vi "Configure RBW List.vi"(8 "error in (no error)":errorcluster, 9 "Resolution Bandwidth Type List":i32[](array[ring])=[0, 0, 0] items=["Gaussian", "Flattop"], 10 "Resolution Bandwidth List":dbl[](array[numeric])=[1000.0, 1000.0, 1000.0], 11 "VISA resource name":refnum<visa-resource-name>) -> (0 "error out":errorcluster, 3 "VISA resource name out":refnum<visa-resource-name>)   [LabVIEW 2018, in "Agilent MXA Series.lvlib"]
doc: "Cofigures the Resolution Bandwidth List under List Sweep measurement type."
uses:
  Agilent MXA Series.lvlib
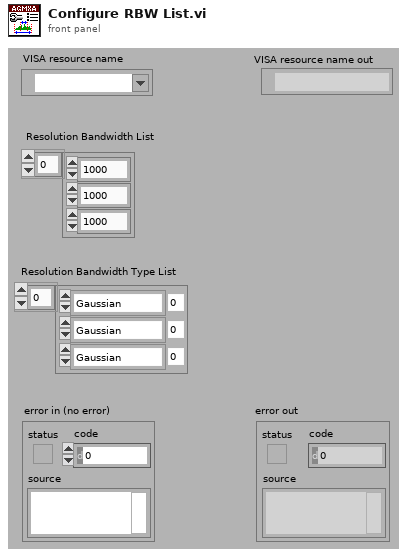
[diagram p1: front panel]
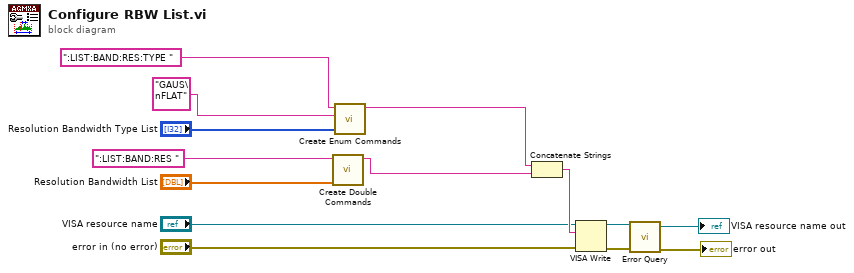
[diagram p0: block diagram]
diagram:
  n1 = call "Create Double Commands.vi"("Double Values"="Resolution Bandwidth List", "Commands"=":LIST:BAND:RES ") -> ("Result"=w5:string)  [unwired: 9 in]
  n2 = call "Create Enum Commands.vi"("Enum Values"="Resolution Bandwidth Type List", "Multi-line Text"="GAUS\nFLAT" ("multi-line string"), "Commands"=":LIST:BAND:RES:TYPE ") -> ("Result"=w1:string)  [unwired: 8 in]
  n3 = Concatenate Strings(w1, w5) -> (w12:string)
  n4 = VISA Write(VISA resource name="VISA resource name", write buffer=w12, error in (no error)="error in (no error)") -> (VISA resource name out=w8:refnum<visa-resource-name>, error out=w9:errorcluster)  [unwired: 1 out]
  n5 = call "Error Query.vi"("error in (no error)"=w9, "VISA resource name"=w8) -> ("error out"=→"error out":errorcluster, "VISA resource name out"=→"VISA resource name out":refnum<visa-resource-name>)  [unwired: 6 in, 2 out]
